vi "VI Span Seite.vi"() -> ()   [LabVIEW 2020, in "FT-IR.lvlib" / "Spanfaktor.lvlib"]
uses:
  Spanfaktor.lvlib
  Visualisierungs Elemente/Zahlen-Ausgabefeld.ctl
  FGV FT-IR Gasliste Aktionen.ctl
  Aktionen EVID-Codes.ctl
  Aktion FGV Span.ctl
  Passwortverwaltung/FGV Passwort Aktion.ctl
  Sprachverwaltung/FGV Aktion Tabelle zerlegen.ctl
  System Einstellungen V2/Aktioen FGV System Konstanten.ctl
  Messdaten/Aktionen FGV Messdaten.ctl
  FGV FT-IR Aktionen.ctl
  Gaszuordnung AO/FGV Gaszuordnung Grenzen&Einheit Aktion.ctl
  Kalibrierung laden.vi
  FT-IR.lvlib
  Messdaten/Messdaten.lvlib
  TOOLweb Interface Library/TOOLweb Interface.lvlib
  Allgemein/allgemeine Sub-VIs.lvlib
  Passwortverwaltung/Passwort.lvlib
  Sprachverwaltung/Sprachverwaltung.lvlib
  Gaszuordnung AO/Gaszuordnung AO.lvlib
  System Einstellungen V2/System Einstellungen V2.lvlib
panel:
  in  "Kalibrierung laden":bool
  in  "in TXT speichern":bool
  in  "Beenden":bool
  in  "Übernehmen":bool[](array[boolean])
  in  "Registerkartenelement":T1(tab)
  in  "Tabelle":string[][](table)
  in  "Average over:":i32=1 caption="Mittelung über:" min=0 max=300 format="%#.0f"
  out "Actual Offset:":T2 caption="Aktueller Offset:" format="%.6f"
  in  "Set new SPAN":bool
  out "Deviation:":T2 caption="Aktual Error:" format="%.2f"
  out "PMwert New Value:":sgl caption="PMwert" format="%.3f"
  out "New Value:":T2 caption="Neue Wert:" format="%.2f"
  out "New SPAN:":T2 caption="Neuer SPAN:" format="%.6f"
  out "Actual SPAN:":T2 caption="Aktueller SPAN:" format="%.6f"
  out "PMwert Actual Value:":sgl caption="PMwert" format="%.3f"
  out "Actual Value:":T2 caption="Aktueller Wert:" format="%.2f"
  out "Einheit":string
  in  "Sollwert":dbl caption="Sollwert:" format="%#.6g"
  in  "Komponente:":u16(ring) items=["NO (350,3000) LP 191C", "NO2 (150) LP 191C (1of2)", "NO2 (2000) LP 191C (2of2)", "N2O (300) LP 191C (1of2)", "NH3 (300) LP 191C (1of2)", "NH3 (900,3000) LP 191C (2of2)", "HNCO (400) 191C", "H2O% (30) LP 191C", "Formaldehyde (70,500) LP 191C", "CO2 low% (4) LP 191C (2of2)", "CO2% (20) LP 191C (1of2)", "CO (700) LP 191C (1of3)", "CO% (1) LP 191C (2of3)", "Propylene (1000) LP 191C", "Aromatic HC C7 (500) LP 191C", "Ethylene (1000) LP 191C", "CH4 (250) LP 191C (1of2)", "CH4 (5000) LP 191C (2of2)", "Ethane (1000) LP 191C", "Acetylene (120) LP 191C", "HNO2 (20) 191C", "MeOH (1000) 191C", "CO% (10) LP 191C (3of3)", "Formic Acid (100) 191C", "SO2 (500) LP 191C", "Acetaldehyde (200) LP 191C", "COS (100) LP 191C", "1,3 butadiene (100) LP 191C", "Oil as Octane (200) LP 191C", "N2O (1000) LP 191C (2of2)"]
  # "Konfiguration Spanfaktoren FT-IR"
  # "Komponente"
  # "Allgemeine Einstellungen"
  # "Aktuelle Werte"
  # "±"
  # "Neue Werte"
  # "±"
  # "sec."
  # "(Wertbereich 1-60 sek.)"
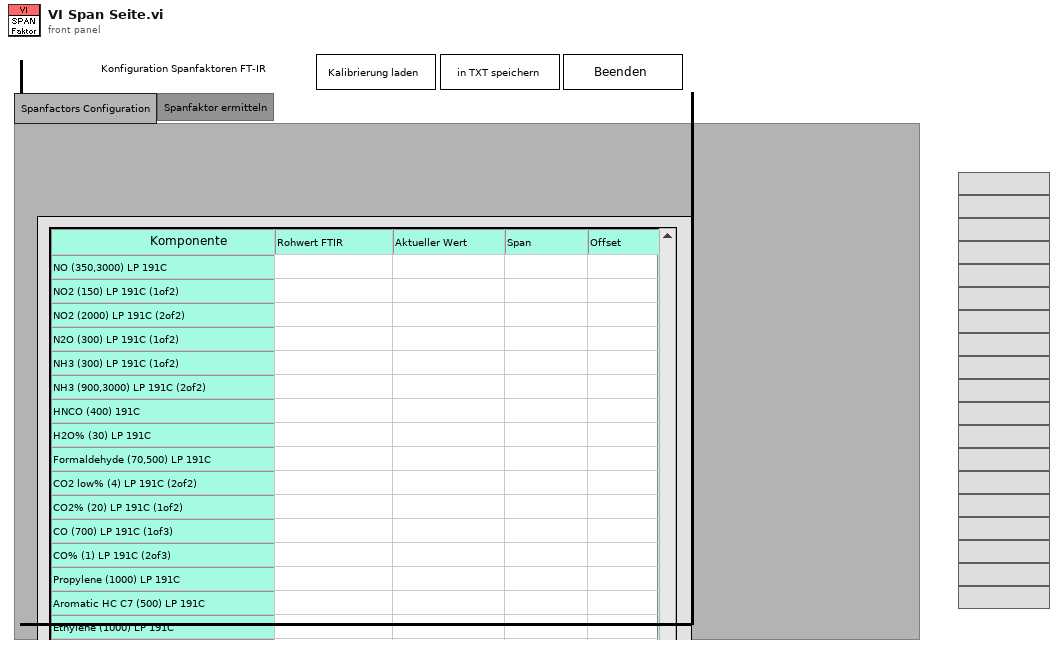
[diagram p1: front panel]
types:
  T1 = enum32{"Spanfactors Configuration", "Determine Spanfactor"}
  T2 = typedef "Zahlen-Ausgabefeld.ctl" = sgl
  T3 = typedef "System Einstellungen V2.lvlib/Aktioen FGV System Konstanten.ctl" = enum16{"lesen", "laden", "speichern", "Sprache"}
  T4 = typedef "Sprachverwaltung.lvlib/FGV Aktion Tabelle zerlegen.ctl" = enum16{"laden", "vereinzeln", "speichern"}
  T5 = typedef "Passwort.lvlib/FGV Passwort Aktion.ctl" = enum16{"prüfen", "setzen", "Initialisieren", "PW speichern", "lesen", "PW Änderung"}
  T6 = typedef "FT-IR.lvlib/Spanfaktor.lvlib/Aktion FGV Span.ctl" = enum16{"lesen", "Span", "Seite aktiv", "Offset", "FGV aktualisiert", "Aktualisierung aufheben"}
  T7 = typedef "FT-IR.lvlib/Aktionen EVID-Codes.ctl" = enum16{"lesen", "setzen", "laden", "speichern", "1Hz/5Hz", "Smoothing", "Rolling Average"}
  T8 = typedef "FT-IR.lvlib/FGV FT-IR Gasliste Aktionen.ctl" = enum16{"lesen", "Gasliste FT-IR", "Gasliste ausgelesen", "laden", "speichern", "löschen"}
  T9 = typedef "String - Ausgabefeld.ctl" = string
  T10 = typedef "FT-IR.lvlib/FGV FT-IR Aktionen.ctl" = enum16{"lesen", "NOG setzen", "NOS setzen", "Initialisieren", "speichern", "ALLES setzen", "FT-IR Spektrum loggen", "Komm Stoppen", "Spektrum LogKonfig"}
  T11 = typedef "Messdaten.lvlib/Aktionen FGV Messdaten.ctl" = enum16{"lesen", "schreiben", "löschen", "Mittelwerte", "Komponente"}
  T12 = typedef "Gaszuordnung AO.lvlib/FGV Gaszuordnung Grenzen&Einheit Aktion.ctl" = enum16{"Lesen", "Schreiben Min", "Schreiben Max", "Laden", "Speichern"}
  T13 = typedef "LVRowAndColumnUnsignedTypeDef.ctl" = cluster{"Row":u32, "Column":u32}
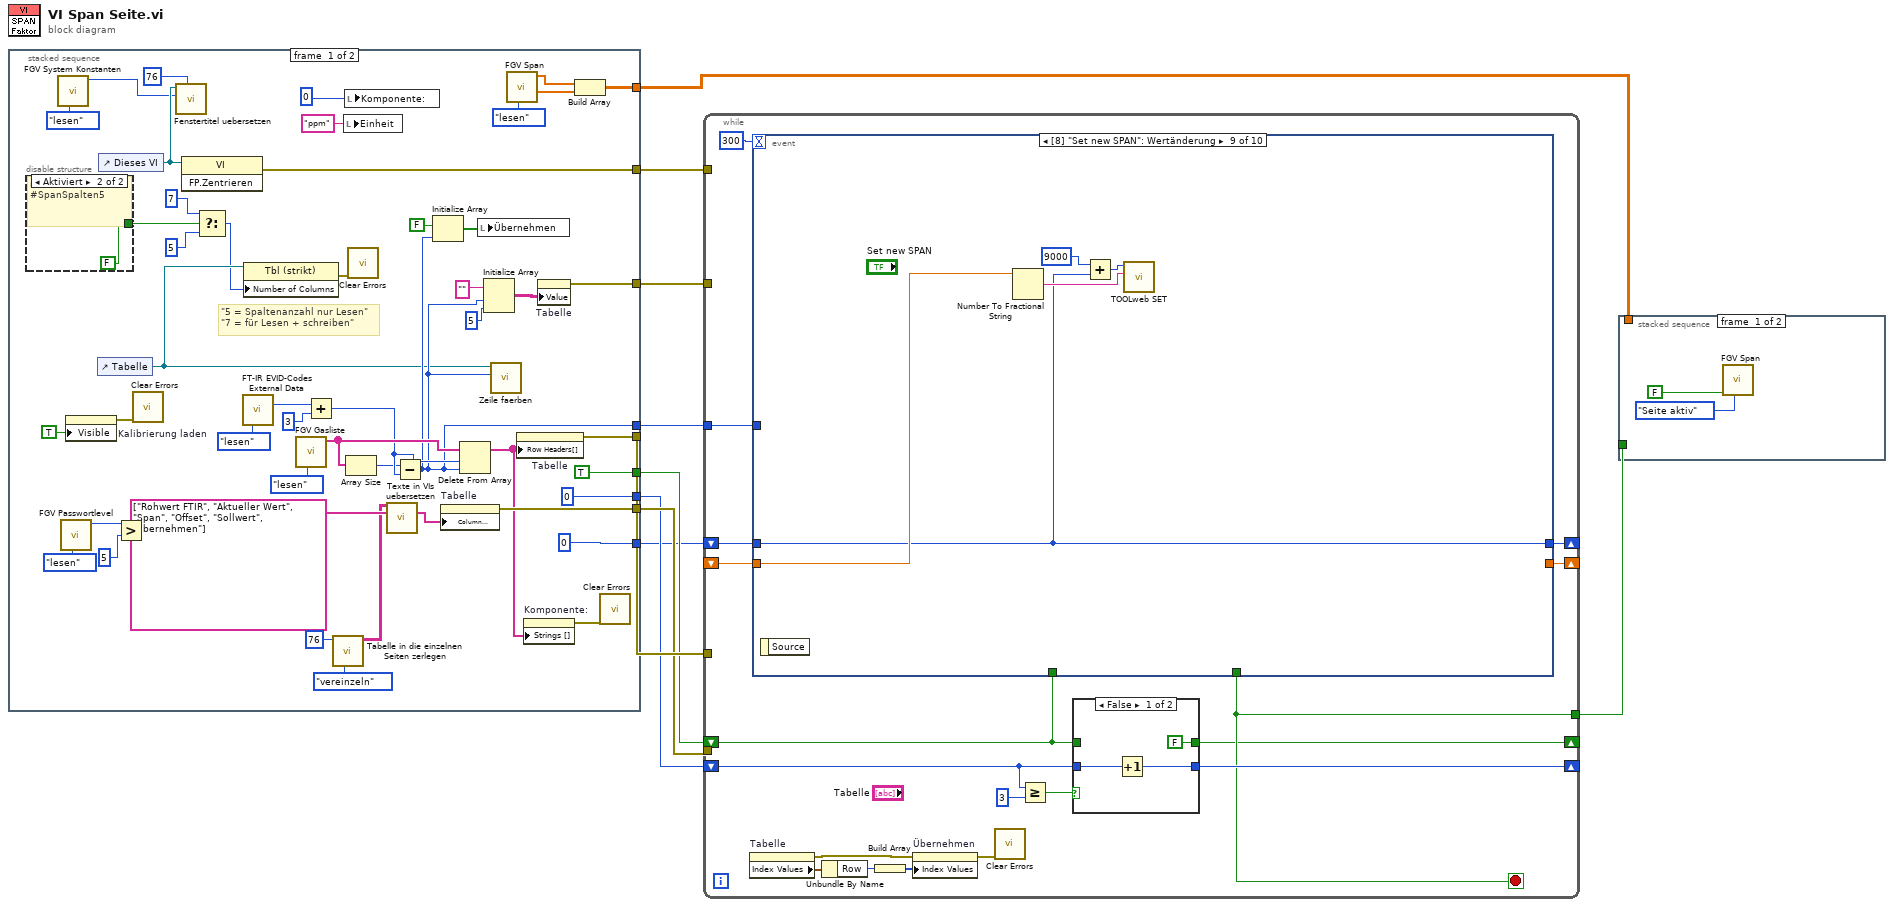
[diagram p0: block diagram]
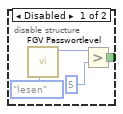
[diagram p2: hidden frame]
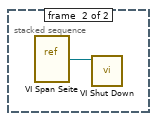
[diagram p4: hidden frame]
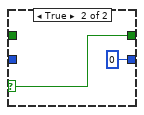
[diagram p5: hidden frame]
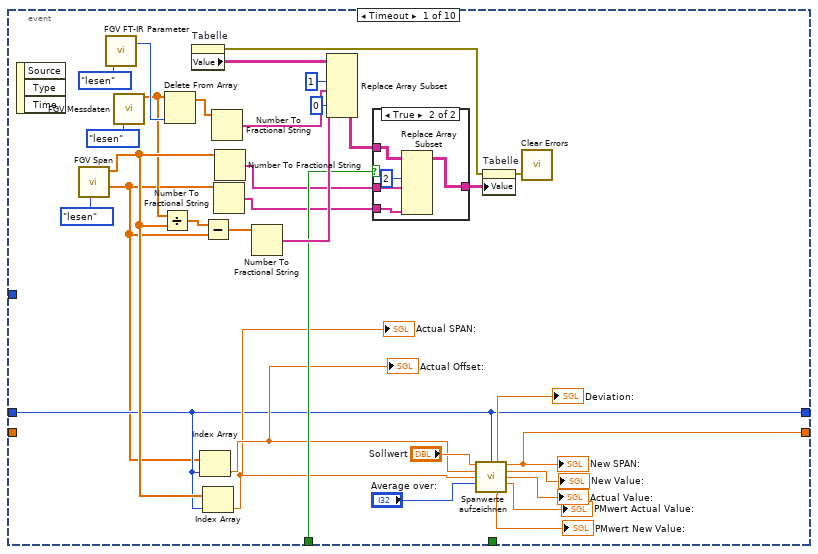
[diagram p6: hidden frame]
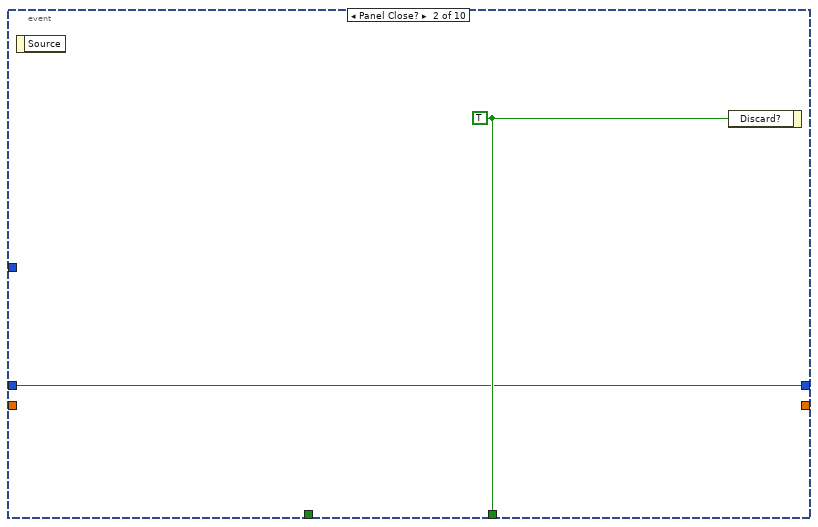
[diagram p8: hidden frame]
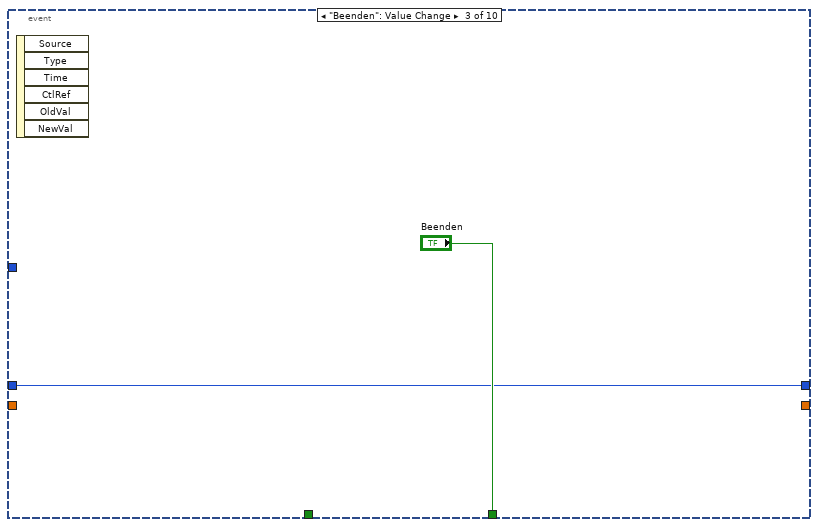
[diagram p9: hidden frame]
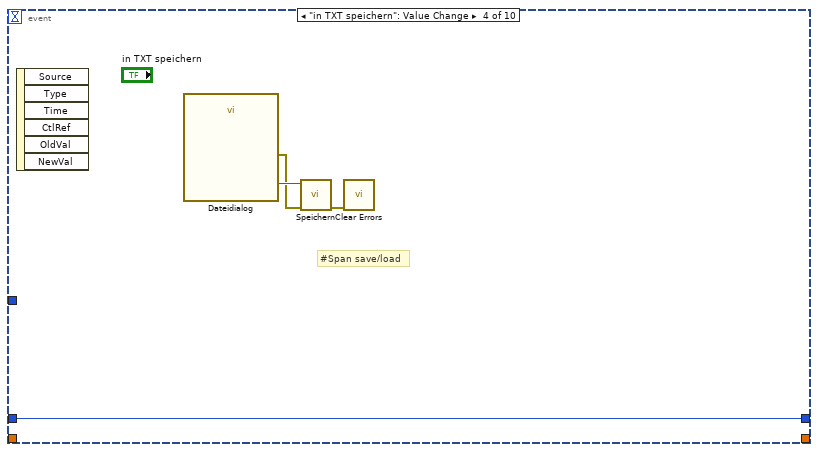
[diagram p10: hidden frame]
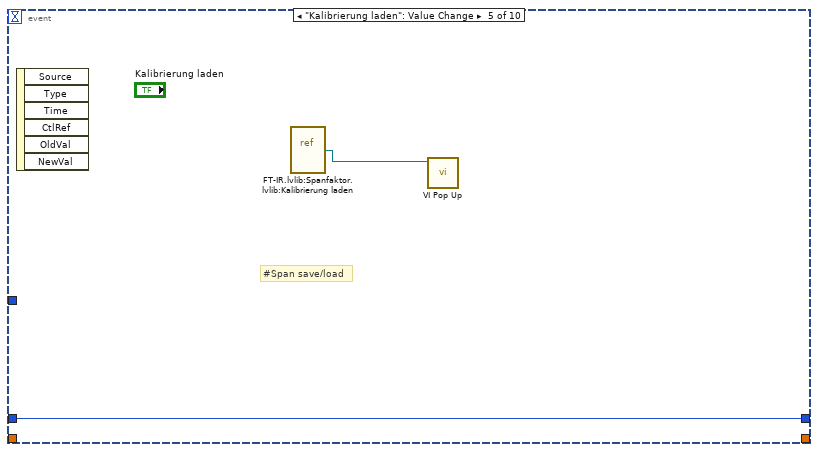
[diagram p11: hidden frame]
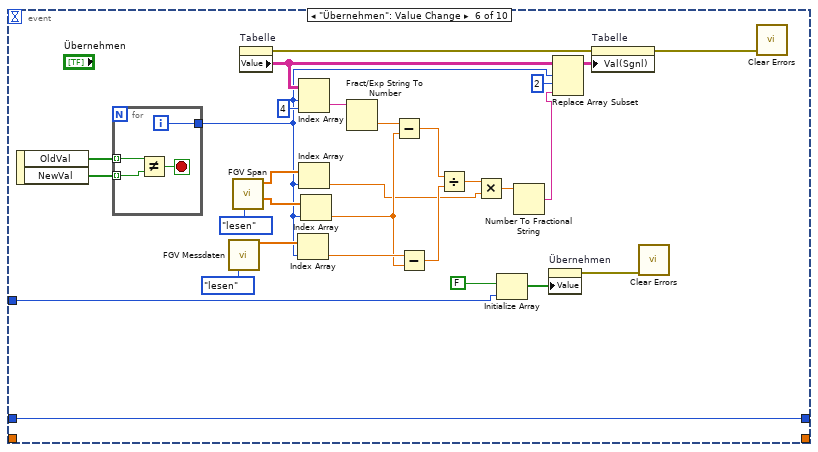
[diagram p12: hidden frame]
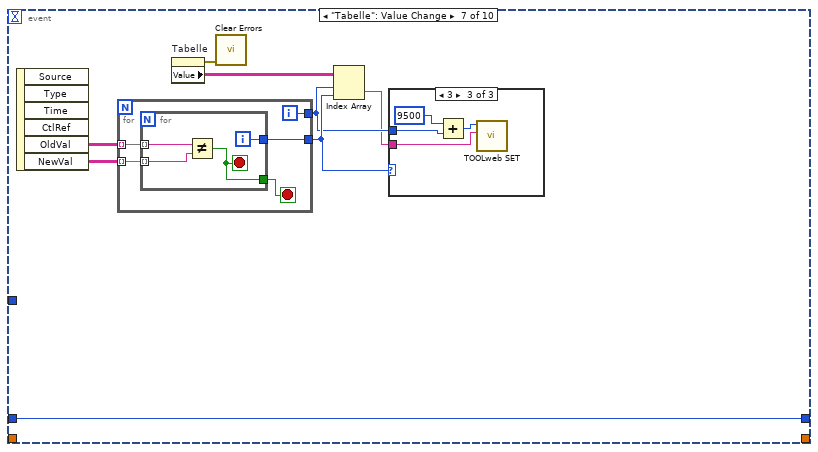
[diagram p13: hidden frame]
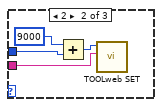
[diagram p15: hidden frame]
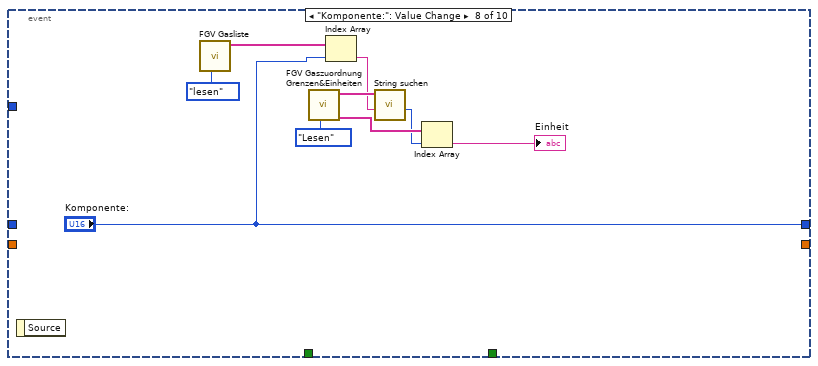
[diagram p16: hidden frame]
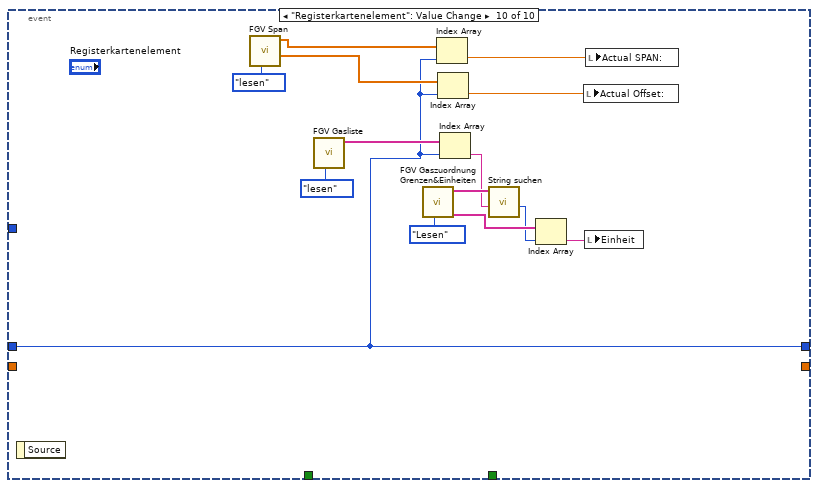
[diagram p17: hidden frame]
diagram:
  n1 = stacked-sequence {
    tunnel: [w58 _] -> w10
    tunnel: [w57 _] -> w9
    tunnel: [0 _] -> w8
    tunnel: [TRUE _] -> w6
    tunnel: [w35 _] -> w5
    tunnel: [w45 _] -> w4
    tunnel: [w42 _] -> w3
    tunnel: [w30 _] -> w2
    tunnel: [u16 0 ("Komponente:") _] -> w1
    frame #0 {
      # "\"5 = Spaltenanzahl nur Lesen\"\n\"7 = für Lesen + schreiben\""
      n2 = disable-structure shown="Aktiviert" {
        disable-tunnel: [w62 FALSE] -> w39
        frame Disabled {
          n3 = call "FGV Passwortlevel.vi"("FGV Passwort Aktion"=FGV_Passwort_Aktion."lesen") -> ("aktueller Level"=w61:i16)  [unwired: 8 in, 2 out]
          n4 = Greater?(x=w61, y=i16 5 ("x")) -> (0:w62:bool)
        }
        frame Enabled {
          # "riw 7.6.18 #SpanSpalten5"
        }
      }
      n5 = call "FGV System Konstanten.vi"("Aktionen"=Aktioen_FGV_System_Konstanten."lesen") -> ("Sprachindex"=w12:u16)  [unwired: 6 in, 4 out]
      n6 = call "FGV Passwortlevel.vi"("FGV Passwort Aktion"=FGV_Passwort_Aktion."lesen") -> ("aktueller Level"=w27:i16)  [unwired: 8 in, 2 out]
      n7 = property on="Kalibrierung laden" class="Bool."("Visible"=TRUE ("Sichtbar")) -> (error out=w26:errorcluster)  [unwired: 2 in, 1 out]
      n8 = control-ref of="Tabelle"() -> (w41:refnum<vi>)
      n9 = control-ref of="Dieses VI"() -> (w19:refnum<vi>)
      n10 = Greater?(x=w27, y=i16 5 ("x")) -> ()  [unwired: 1 out]
      n11 = call <vilib>:"Clear Errors.vi"("error in (no error)"=w26) -> ()  [unwired: 5 in, 2 out]
      n12 = call "Fenstertitel uebersetzen.vi"("Index (Seite)"=u16 76 ("Sprachauswahl"), "Sprachauswahl"=w12, "Dieses VI"=w19) -> ()  [unwired: 5 in, 4 out]
      n13 = invoke class="VI" method="FP.Zentrieren"(reference=w19) -> (error out=w45:errorcluster)  [unwired: 2 in, 2 out]
      n14 = Select(t=u32 7, s=w39, f=u32 5) -> (s? t:f=w36:u32)
      n15 = call "FT-IR EVID-Codes External Data.vi"("Aktionen"=Aktionen_EVID-Codes."lesen") -> ("Anzahl"=w53:i32)  [unwired: 9 in, 5 out]
      n16 = property class="Tbl (strikt)"(reference=w41, "Number of Columns"=w36) -> (error out=w40:errorcluster)  [unwired: 1 in, 1 out]
      n17 = call "FGV Gasliste.vi"("Aktionen"=FGV_FT-IR_Gasliste_Aktionen."lesen") -> ("Aktuelle Gasliste FT-IR"=w51:T9[])  [unwired: 8 in, 2 out]
      n18 = Add(x=w53, y=3) -> (x+y=w50:i32)
      n19 = call "Tabelle in die einzelnen Seiten zerlegen.vi"("Aktion"=FGV_Aktion_Tabelle_zerlegen."vereinzeln", "Index (Seite)"=76) -> ("Sprachliste"=w20:string[][])  [unwired: 7 in, 2 out]
      n20 = local write "Einheit"("ppm" ("Einheit")) -> ()
      n21 = local write "Komponente:"(u16 0 ("Komponente:")) -> ()
      n22 = Array Size(array=w51) -> (size(s)=w49:i32)
      n23 = call <vilib>:"Clear Errors.vi"("error in (no error)"=w40) -> ()  [unwired: 5 in, 2 out]
      n24 = call "Texte in VIs uebersetzen.vi"("Sprachliste"=w20, "String-Array zum Übersetzen"=string[] ["Rohwert FTIR", "Aktueller Wert", "Span", "Offset", "Sollwert", "übernehmen"] ("Spaltentitel[]")) -> ("String-Array zum Übersetzen"=w21:string[])  [unwired: 9 in, 4 out]
      n25 = Subtract(x=w49, y=w50) -> (x-y=w42:i32)
      n26 = Initialize Array(FALSE, w42) -> (w43:bool[])
      n27 = property on="Tabelle" class="Tbl (strikt)"("Column Headers[]"=w21) -> (error out=w57:errorcluster)  [unwired: 2 in, 1 out]
      n28 = Delete From Array(array=w51, length=w50, index=w42) -> (array with subset deleted=w17:T9[])  [unwired: 1 out]
      n29 = local write "Übernehmen"(w43) -> ()
      n30 = Initialize Array("", w42, 5 ("Dimension")) -> (w34:string[][])
      n31 = call "Zeile faerben.vi"("Anzahl"=w42, "Table (Eingang)"=w41) -> ()  [unwired: 9 in, 1 out]
      n32 = call "FGV Span.vi"("Aktion"=Aktion_FGV_Span."lesen") -> ("Offset"=w31:sgl[], "Span"=w32:sgl[])  [unwired: 7 in, 2 out]
      n33 = property on="Tabelle" class="Tbl (strikt)"("Row Headers[]"=w17) -> (error out=w58:errorcluster)  [unwired: 2 in, 1 out]
      n34 = property on="Komponente:" class="Ring (strikt)"("Strings []"=w17) -> (error out=w16:errorcluster)  [unwired: 2 in, 1 out]
      n35 = property on="Tabelle" class="Tbl (strikt)"("Value"=w34) -> (error out=w35:errorcluster)  [unwired: 2 in, 1 out]
      n36 = Build Array(w32, w31) -> (w30:sgl[][])
      n37 = call <vilib>:"Clear Errors.vi"("error in (no error)"=w16) -> ()  [unwired: 5 in, 2 out]
    }
    frame #1 {
    }
  }
  n38 = while {
    tunnel: w10 -> [_]
    tunnel: w9 -> [_]
    shift-right: [w77] -> _
    shift-left: w8 -> [w79]
    tunnel: [w76] -> w7
    shift-right: [w75] -> _
    shift-left: w6 -> [w74]
    tunnel: w5 -> [_]
    tunnel: w4 -> [_]
    tunnel: w3 -> [w68]
    shift-right: [w67] -> _
    shift-left: w1 -> [w66]
    shift-right: [w65] -> _
    shift-left: _ -> [w64]
    stop <- w76 stop-if-true
    n39 = property on="Tabelle" class="Tbl (strikt)"() -> (error out=w70:errorcluster, "Index Values"=w71:T13)  [unwired: 2 in, 1 out]
    n40 = event shown="[8] \"Set new SPAN\": Wertänderung" {
      selector: _ -> [_ _ _ _ _ _ _ _ _ _]
      dyn-events: _ -> [_ _ _ _ _ _ _ _ _ _]
      timeout: 300 -> [_ _ _ _ _ _ _ _ _ _]
      tunnel: w74 -> [w107 _ _ _ _ _ _ _ _ _]
      tunnel: [_ w127 "Beenden" _ _ _ _ _ _ _] -> w76
      tunnel: w68 -> [_ _ _ _ _ w140 _ _ _ _]
      tunnel: [w90 w126 w128 w130 w134 w136 w169 "Komponente:" w203 w211] -> w67
      tunnel: w66 -> [w90 w126 w128 w130 w134 w136 w169 _ w203 w211]
      tunnel: [w99 _ _ _ _ _ _ _ _ _] -> w65
      tunnel: w64 -> [_ _ _ _ _ _ _ _ w205 _]
      event Timeout {
        n41 = event-data() -> ()  [unwired: 1 in, 3 out]
        n42 = call "FGV Span.vi"("Aktion"=Aktion_FGV_Span."lesen") -> ("Offset"=w87:sgl[], "Span"=w94:sgl[])  [unwired: 7 in, 2 out]
        n43 = call "FGV FT-IR Parameter.vi"("Aktion"=FGV_FT-IR_Aktionen."lesen") -> ("NoOfGasses"=w93:u32)  [unwired: 11 in, 7 out]
        n44 = call "FGV Messdaten.vi"("Aktionen"=Aktionen_FGV_Messdaten."lesen") -> ("Aktuelle Messwerte"=w89:sgl[])  [unwired: 6 in, 8 out]
        n45 = Divide(x=w89, y=w94) -> (x/y=w110:sgl[])
        n46 = Delete From Array(array=w89, index=w93) -> (array with subset deleted=w111:sgl[])  [unwired: 1 in, 1 out]
        n47 = property on="Tabelle" class="Tbl (strikt)"() -> (error out=w104:errorcluster, "Value"=w116:string[][])  [unwired: 2 in, 1 out]
        n48 = Index Array(array=w87, index=w90) -> (element=w92:sgl)
        "Actual Offset:" <- w92
        n49 = Subtract(x=w110, y=w87) -> (x-y=w88:sgl[])
        n50 = Index Array(array=w94, index=w90) -> (element=w91:sgl)
        "Actual SPAN:" <- w91
        n51 = Number To Fractional String(number=w111) -> (F-format string=w114:string[])  [unwired: 3 in]
        n52 = Number To Fractional String(number=w87) -> (F-format string=w105:string[])  [unwired: 3 in]
        n53 = Number To Fractional String(number=w94) -> (F-format string=w106:string[])  [unwired: 3 in]
        n54 = Number To Fractional String(number=w88) -> (F-format string=w113:string[])  [unwired: 3 in]
        n55 = Replace Array Subset(array=w116, new element #1=w114, index (col) #1=1 ("Deaktivierter Index (Spalte)"), new element #2=w113, index (col) #2=0 ("Index (Spalte)")) -> (w109:string[][])  [unwired: 2 in]
        n56 = case shown="True" w107 {
          tunnel: w109 -> [w120 w125]
          tunnel: [w120 w124] -> w108
          tunnel: w106 -> [_ w123]
          tunnel: w105 -> [_ w122]
          frame False {
          }
          frame True {
            n57 = Replace Array Subset(array=w125, new element #1=w123, index (col) #1=2 ("Deaktivierter Index (Spalte)"), new element #2=w122) -> (w124:string[][])  [unwired: 3 in]
          }
        }
        n58 = call "Spanwerte aufzeichnen.vi"("Sollwerte"="Sollwert", "Komponente"=w90, "Offset"=w92, "Aktueller Spanfactor"=w91, "Mittelung in sec"="Average over:") -> ("Aktuelle Fehler"=→"Deviation:":sgl, "Spanfaktor"=w99:sgl, "Neuer Wert"=→"New Value:":sgl, "Aktueller Wert gemittelt"=→"Actual Value:":sgl, "Aktuelle Standardabweichung"=→"PMwert Actual Value:":sgl, "neue Standardabweichung"=→"PMwert New Value:":sgl)  [unwired: 4 in, 1 out]
        "New SPAN:" <- w99
        n59 = property on="Tabelle" class="Tbl (strikt)"(error in=w104, "Value"=w108) -> (error out=w103:errorcluster)  [unwired: 1 in, 1 out]
        n60 = call <vilib>:"Clear Errors.vi"("error in (no error)"=w103) -> ()  [unwired: 5 in, 2 out]
      }
      event Panel Close? {
        w127 = TRUE ("Verwerfen?")
        n61 = event-data() -> ()  [unwired: 1 in, 1 out]
        n62 = event-data("Discard?"=w127) -> ()  [unwired: 1 in, 1 out]
      }
      event "Beenden": Value Change {
        n63 = event-data() -> ()  [unwired: 1 in, 6 out]
      }
      event "in TXT speichern": Value Change {
        # "#Span save/load"
        n64 = event-data() -> ()  [unwired: 1 in, 6 out]
        n65 = call "Dateidialog"() -> ("selected path"=w132:path, "error out"=w131:errorcluster)  [unwired: 12 in, 2 out]
        n66 = call "Speichern.vi"("Fehler (Eingang)"=w131, "pfad"=w132) -> ("Fehler (Ausgang)"=w133:errorcluster)  [unwired: 9 in]
        n67 = call <vilib>:"Clear Errors.vi"("error in (no error)"=w133) -> ()  [unwired: 5 in, 2 out]
      }
      event "Kalibrierung laden": Value Change {
        # "#Span save/load"
        n68 = event-data() -> ()  [unwired: 1 in, 6 out]
        n69 = vi-ref "FT-IR.lvlib:Spanfaktor.lvlib:Kalibrierung laden.vi"() -> (w135:refnum<vi>)
        n70 = call "VI Pop Up.vi"("VI Referenz"=w135) -> ()  [unwired: 10 in, 1 out]
      }
      event "Übernehmen": Value Change {
        n71 = event-data() -> ("OldVal"=w164:bool[], "NewVal"=w163:bool[])  [unwired: 1 in]
        n72 = for {
          tunnel: w164 -> [w168] mode=indexing
          tunnel: w163 -> [w167] mode=indexing
          tunnel: [w165] -> w137
          i -> [w165]
          stop <- w166 stop-if-true
          n73 = Not Equal?(x=w168, y=w167) -> (x != y?=w166:bool)
        }
        n74 = call "FGV Messdaten.vi"("Aktionen"=Aktionen_FGV_Messdaten."lesen") -> ("Aktuelle Messwerte"=w155:sgl[])  [unwired: 6 in, 8 out]
        n75 = call "FGV Span.vi"("Aktion"=Aktion_FGV_Span."lesen") -> ("Offset"=w158:sgl[], "Span"=w159:sgl[])  [unwired: 7 in, 2 out]
        n76 = property on="Tabelle" class="Tbl (strikt)"() -> (error out=w143:errorcluster, "Value"=w147:string[][])  [unwired: 2 in, 1 out]
        n77 = Index Array(array=w155, index=w137) -> (element=w154:sgl)
        n78 = Index Array(array=w147, index (row)=w137, index (col)=4 ("Deaktivierter Index (Spalte)")) -> (element=w161:string)
        n79 = Index Array(array=w159, index=w137) -> (element=w149:sgl)
        n80 = Index Array(array=w158, index=w137) -> (element=w153:sgl)
        n81 = Fract/Exp String To Number(string=w161) -> (number=w157:dbl)  [unwired: 3 in, 1 out]
        n82 = Subtract(x=w157, y=w153) -> (x-y=w152:dbl)
        n83 = Subtract(x=w154, y=w153) -> (x-y=w151:sgl)
        n84 = Divide(x=w152, y=w151) -> (x/y=w150:dbl)
        n85 = Multiply(x=w150, y=w149) -> (x*y=w148:dbl)
        n86 = Initialize Array(FALSE, w140) -> (w139:bool[])
        n87 = Number To Fractional String(number=w148) -> (F-format string=w144:string)  [unwired: 3 in]
        n88 = property on="Übernehmen" class="Arr"("Value"=w139) -> (error out=w138:errorcluster)  [unwired: 2 in, 1 out]
        n89 = Replace Array Subset(array=w147, new element=w144, index (row)=w137, index (col)=2 ("Deaktivierter Index (Spalte)")) -> (w146:string[][])
        n90 = property on="Tabelle" class="Tbl (strikt)"(error in=w143, "Val(Sgnl)"=w146) -> (error out=w142:errorcluster)  [unwired: 1 in, 1 out]
        n91 = call <vilib>:"Clear Errors.vi"("error in (no error)"=w138) -> ()  [unwired: 5 in, 2 out]
        n92 = call <vilib>:"Clear Errors.vi"("error in (no error)"=w142) -> ()  [unwired: 5 in, 2 out]
      }
      event "Tabelle": Value Change {
        n93 = event-data() -> ("OldVal"=w176:string[][], "NewVal"=w175:string[][])  [unwired: 1 in, 4 out]
        n94 = for {
          tunnel: w176 -> [w187] mode=indexing
          tunnel: w175 -> [w186] mode=indexing
          tunnel: [w189] -> w172
          tunnel: [w188] -> w173
          i -> [w189]
          stop <- w185 stop-if-true
          n95 = for {
            tunnel: w186 -> [w192] mode=indexing
            tunnel: w187 -> [w193] mode=indexing
            tunnel: [w191] -> w188
            tunnel: [w190] -> w185
            i -> [w191]
            stop <- w190 stop-if-true
            n96 = Not Equal?(x=w193, y=w192) -> (x != y?=w190:bool)
          }
        }
        n97 = property on="Tabelle" class="Tbl (strikt)"() -> (error out=w170:errorcluster, "Value"=w174:string[][])  [unwired: 2 in, 1 out]
        n98 = call <vilib>:"Clear Errors.vi"("error in (no error)"=w170) -> ()  [unwired: 5 in, 2 out]
        n99 = Index Array(array=w174, index (row)=w172, index (col)=w173) -> (element=w171:string)
        n100 = case shown="3" w173 {
          tunnel: w172 -> [_ w178 w182]
          tunnel: w171 -> [_ w177 w181]
          frame 0, Default {
          }
          frame 2 {
            n101 = Add(x=9000 ("Feedback"), y=w178) -> (x+y=w180:i32)
            n102 = call "TOOLweb SET.vi"("Wert-String"=w177, "EVID-Nummer"=w180) -> ()  [unwired: 3 in, 3 out]
          }
          frame 3 {
            n103 = Add(x=9500 ("Feedback"), y=w182) -> (x+y=w184:i32)
            n104 = call "TOOLweb SET.vi"("Wert-String"=w181, "EVID-Nummer"=w184) -> ()  [unwired: 3 in, 3 out]
          }
        }
      }
      event "Komponente:": Value Change {
        n105 = event-data() -> ()  [unwired: 1 in, 1 out]
        n106 = call "FGV Gasliste.vi"("Aktionen"=FGV_FT-IR_Gasliste_Aktionen."lesen") -> ("Aktuelle Gasliste FT-IR"=w202:T9[])  [unwired: 8 in, 2 out]
        n107 = call "FGV Gaszuordnung Grenzen&Einheiten.vi"("Aktion"=FGV_Gaszuordnung_Grenzen&Einheit_Aktion."Lesen") -> ("Einheit neu"=w199:string[], "Namen neu"=w198:string[])  [unwired: 7 in, 2 out]
        n108 = Index Array(array=w202, index="Komponente:") -> (element=w196:T9)
        n109 = call "String suchen.vi"("Gasname"=w196, "Such-Namen"=w198) -> ("Index"=w197:i32)  [unwired: 8 in, 1 out]
        n110 = Index Array(array=w199, index=w197) -> (element=→"Einheit":string)
      }
      event "Set new SPAN": Value Change {
        n111 = event-data() -> ()  [unwired: 1 in, 1 out]
        n112 = Number To Fractional String(number=w205) -> (F-format string=w204:string)  [unwired: 3 in]
        n113 = Add(x=9000 ("Feedback"), y=w203) -> (x+y=w207:i32)
        n114 = call "TOOLweb SET.vi"("Wert-String"=w204, "EVID-Nummer"=w207) -> ()  [unwired: 3 in, 3 out]
      }
      event "Registerkartenelement": Value Change {
        n115 = event-data() -> ()  [unwired: 1 in, 1 out]
        n116 = call "FGV Span.vi"("Aktion"=Aktion_FGV_Span."lesen") -> ("Offset"=w212:sgl[], "Span"=w213:sgl[])  [unwired: 7 in, 2 out]
        n117 = call "FGV Gasliste.vi"("Aktionen"=FGV_FT-IR_Gasliste_Aktionen."lesen") -> ("Aktuelle Gasliste FT-IR"=w221:T9[])  [unwired: 8 in, 2 out]
        n118 = call "FGV Gaszuordnung Grenzen&Einheiten.vi"("Aktion"=FGV_Gaszuordnung_Grenzen&Einheit_Aktion."Lesen") -> ("Einheit neu"=w218:string[], "Namen neu"=w217:string[])  [unwired: 7 in, 2 out]
        n119 = Index Array(array=w213, index=w211) -> (element=w210:sgl)
        n120 = Index Array(array=w212, index=w211) -> (element=w209:sgl)
        n121 = Index Array(array=w221, index=w211) -> (element=w215:T9)
        n122 = call "String suchen.vi"("Gasname"=w215, "Such-Namen"=w217) -> ("Index"=w216:i32)  [unwired: 8 in, 1 out]
        n123 = Index Array(array=w218, index=w216) -> (element=w208:string)
        n124 = local write "Actual Offset:"(w209) -> ()
        n125 = local write "Einheit"(w208) -> ()
        n126 = local write "Actual SPAN:"(w210) -> ()
      }
    }
    n127 = Unbundle By Name(w71) -> ("Row"=w72:u32)
    n128 = Build Array(w72) -> (w73:u32[])
    n129 = property on="Übernehmen" class="Arr"(error in=w70, "Index Values"=w73) -> (error out=w69:errorcluster)  [unwired: 1 in, 1 out]
    n130 = call <vilib>:"Clear Errors.vi"("error in (no error)"=w69) -> ()  [unwired: 5 in, 2 out]
    n131 = Greater Or Equal?(x=w79, y=3) -> (x >= y?=w78:bool)
    n132 = case shown="False" w78 {
      selector: w78 -> [_ w85]
      tunnel: w79 -> [w84 _]
      tunnel: [w83 0] -> w77
      tunnel: [FALSE w85] -> w75
      tunnel: w74 -> [_ _]
      frame False {
        n133 = Increment(x=w84) -> (x+1=w83:i32)
      }
      frame True {
      }
    }
  }
  n134 = stacked-sequence {
    tunnel: w7 -> [_ _]
    tunnel: w2 -> [_ _]
    frame #0 {
      n135 = call "FGV Span.vi"("Aktion"=Aktion_FGV_Span."Seite aktiv", "Aktiv"=FALSE) -> ()  [unwired: 6 in, 4 out]
    }
    frame #1 {
      n136 = vi-ref "VI Span Seite.vi"() -> (w224:refnum<vi>)
      n137 = call "VI Shut Down.vi"("VI Referenz"=w224) -> ()  [unwired: 11 in]
    }
  }
